vi "Update Current Segment.vi"(8 "error in (no error)":errorcluster, 10 "Waveform Size":i32, 11 "Waveform Buffer in":refnum<class "Waveform Buffer.lvclass">) -> (0 "error out":errorcluster, 3 "Waveform Buffer out":refnum<class "Waveform Buffer.lvclass">)   [LabVIEW 2015, in "Waveform Buffer.lvclass"]
uses:
  Waveform Buffer.lvclass
  Waveform Buffer.lvclass/Waveform Buffer.ctl
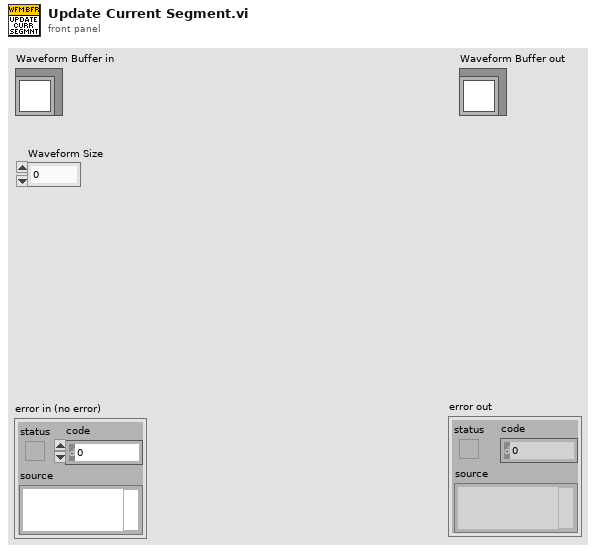
[diagram p1: front panel]
types:
  T1 = typedef "Waveform Buffer.lvclass/Wfm Segment.ctl" = cluster{"ID":u64, "Total samples":i32, "Start":T2, "Finish":T2}
  T2 = typedef "Waveform Buffer.lvclass/Data Point.ctl" = cluster{"Index":i32, "Wfm time":timestamp, "Receive time":timestamp}
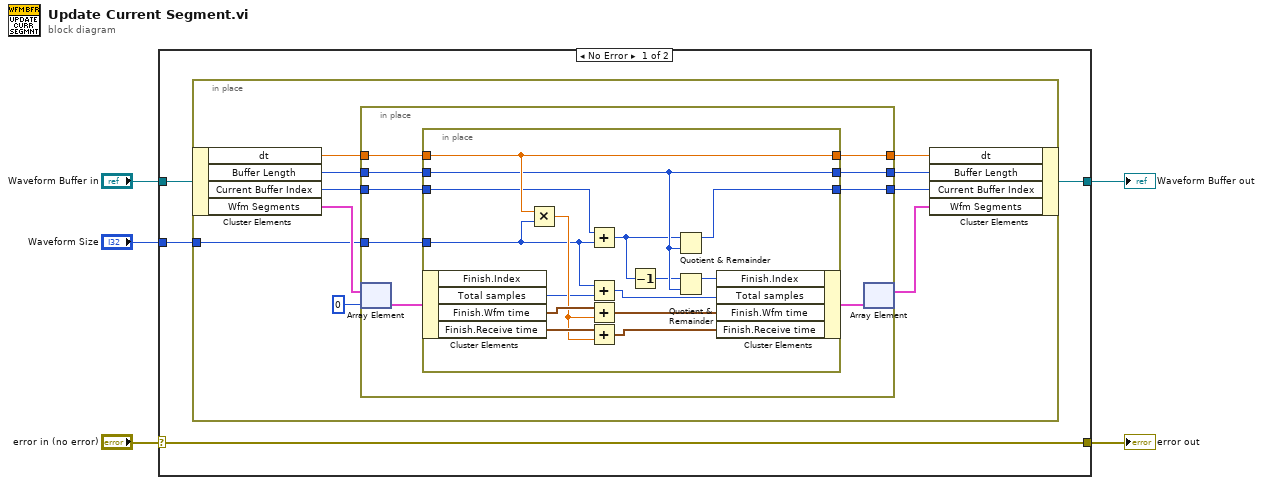
[diagram p0: block diagram]
diagram:
  n1 = case shown="No Error" "error in (no error)" {
    selector: "error in (no error)" -> [w9 w45]
    tunnel: [w9 w45] -> w4
    tunnel: [w6 w44] -> w3
    tunnel: "Waveform Buffer in" -> [w8 w44]
    tunnel: "Waveform Size" -> [w7 _]
    frame No Error {
      n2 = in-place {
        in-place-border: w7 -> [w12]
        n3 = in-place-cluster #1(w8) -> ("dt"=w16:dbl, "Buffer Length"=w15:i32, "Current Buffer Index"=w13:i32, "Wfm Segments"=w19:T1[])
        n4 = in-place {
          in-place-border: [w27] -> w17
          in-place-border: w16 -> [w26]
          in-place-border: w15 -> [w25]
          in-place-border: [w24] -> w14
          in-place-border: w13 -> [w23]
          in-place-border: w12 -> [w22]
          in-place-border: [w21] -> w11
          n5 = in-place-array #2(w19, 0) -> (w28:T1)
          n6 = in-place {
            in-place-border: [w43] -> w27
            in-place-border: w26 -> [w43]
            in-place-border: w25 -> [w33]
            in-place-border: [w33] -> w24
            in-place-border: w23 -> [w34]
            in-place-border: w22 -> [w29]
            in-place-border: [w35] -> w21
            n7 = in-place-cluster #3(w28) -> ("Total samples"=w37:i32, "Finish.Wfm time"=w42:timestamp, "Finish.Receive time"=w40:timestamp)  [unwired: 1 out]
            n8 = Multiply(x=w43, y=w29) -> (x*y=w38:dbl)
            n9 = Add(x=w34, y=w29) -> (x+y=w32:i32)
            n10 = Add(x=w29, y=w37) -> (x+y=w36:i32)
            n11 = Add(x=w42, y=w38) -> (x+y=w41:timestamp)
            n12 = Add(x=w40, y=w38) -> (x+y=w39:timestamp)
            n13 = Decrement(x=w32) -> (x-1=w31:i32)
            n14 = Quotient & Remainder(x=w32, y=w33) -> (x-y*floor(x/y)=w35:i32)  [unwired: 1 out]
            n15 = Quotient & Remainder(x=w31, y=w33) -> (x-y*floor(x/y)=w30:i32)  [unwired: 1 out]
            n16 = in-place-cluster #3("Finish.Index"=w30, "Total samples"=w36, "Finish.Wfm time"=w41, "Finish.Receive time"=w39) -> (w20:T1)
          }
          n17 = in-place-array #2(w20) -> (w10:T1[])  [unwired: 1 out]
        }
        n18 = in-place-cluster #1("dt"=w17, "Buffer Length"=w14, "Current Buffer Index"=w11, "Wfm Segments"=w10) -> (w6:refnum<class "Waveform Buffer.lvclass">)
      }
    }
    frame Error {
    }
  }
  "error out" <- w4
  "Waveform Buffer out" <- w3
